vi "semaphor.vi"() -> ()   [LabVIEW 2020]
panel:
  out "x+y":i32
  out "error out 2":errorcluster
  out "error out":errorcluster
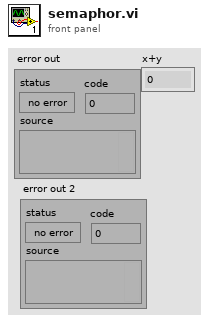
[diagram p1: front panel]
types:
  T1 = typedef "Semaphore RefNum" = refnum<k1>
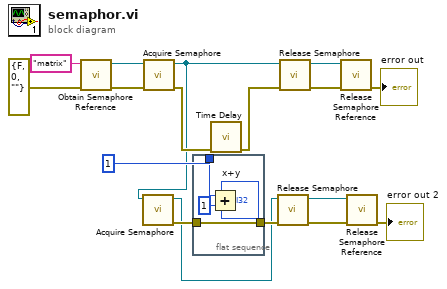
[diagram p0: block diagram]
diagram:
  n1 = call <vilib>:"Obtain Semaphore Reference.vi"("error in (no error)"=errorcluster {"status"=FALSE, "code"=0, "source"=""}, "name (unnamed)"="matrix") -> ("error out"=w13:errorcluster, "semaphore"=w12:T1)  [unwired: 3 in, 1 out]
  n2 = call <vilib>:"Acquire Semaphore.vi"("error in (no error)"=w13, "semaphore"=w12) -> ("error out"=w14:errorcluster, "semaphore out"=w1:T1)  [unwired: 3 in, 1 out]
  n3 = call <vilib>:"Acquire Semaphore.vi"("semaphore"=w1) -> ("error out"=w4:errorcluster, "semaphore out"=w2:T1)  [unwired: 4 in, 1 out]
  n4 = flat-sequence {
    tunnel: [w21] -> w5
    tunnel: w4 -> [w21]
    tunnel: 1 -> [w20]
    frame #0 {
      n5 = Add(x=w20, y=1) -> (x+y=→"x+y":i32)
    }
  }
  n6 = call "Time Delay"("error in (no error)"=w14) -> ("error out"=w15:errorcluster)  [unwired: 10 in]
  n7 = call <vilib>:"Release Semaphore.vi"("error in (no error)"=w5, "semaphore"=w2) -> ("error out"=w8:errorcluster, "semaphore out"=w7:T1)  [unwired: 4 in]
  n8 = call <vilib>:"Release Semaphore.vi"("error in (no error)"=w15, "semaphore"=w1) -> ("error out"=w17:errorcluster, "semaphore out"=w16:T1)  [unwired: 4 in]
  n9 = call <vilib>:"Release Semaphore Reference.vi"("error in (no error)"=w17, "semaphore"=w16) -> ("error out"=→"error out":errorcluster)  [unwired: 8 in, 1 out]
  n10 = call <vilib>:"Release Semaphore Reference.vi"("error in (no error)"=w8, "semaphore"=w7) -> ("error out"=→"error out 2":errorcluster)  [unwired: 8 in, 1 out]
